vi "Random Color Generator.vi"(5 "Lightest Limit":u32(colorbox)=16448250, 7 "Darkest Limit":u32(colorbox), 11 "Color Exclude":u32[](array[colorbox])) -> (1 "Random Color":u32(colorbox), 3 "Color Exclude Out":u32[](array[numeric]))   [LabVIEW 2023]
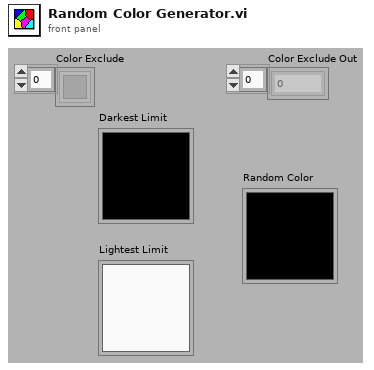
[diagram p1: front panel]
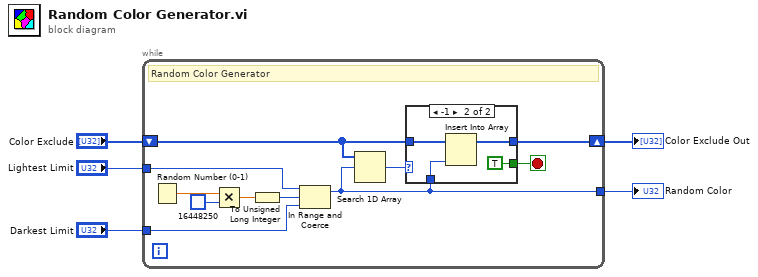
[diagram p0: block diagram]
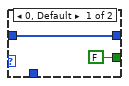
[diagram p2: hidden frame]
diagram:
  n1 = while {
    tunnel: "Darkest Limit" -> [w14]
    tunnel: "Lightest Limit" -> [w13]
    tunnel: [w8] -> w3
    shift-right: [w9] -> w1
    shift-left: "Color Exclude" -> [w10]
    stop <- w6 stop-if-true
    # "Random Color Generator"
    n2 = Random Number (0-1)() -> (number: 0 to 1=w16:dbl)
    n3 = Multiply(x=w16, y=u32 16448250 ("Lightest Limit 2")) -> (x*y=w12:dbl)
    n4 = To Unsigned Long Integer(number=w12) -> (unsigned 32bit integer=w11:u32)
    n5 = In Range and Coerce(upper limit=w13, x=w11, lower limit=w14) -> (coerced(x)=w8:u32)  [unwired: 1 out]
    n6 = Search 1D Array(1D array=w10, element=w8) -> (index of element=w7:i32)  [unwired: 1 in]
    n7 = case shown="-1" w7 {
      tunnel: w10 -> [w17 w22]
      tunnel: [w17 w21] -> w9
      tunnel: w8 -> [_ w20]
      tunnel: [FALSE TRUE] -> w6
      frame 0, Default {
      }
      frame -1 {
        n8 = Insert Into Array(array=w22, new element=w20) -> (w21:u32[])  [unwired: 1 in]
      }
    }
  }
  "Random Color" <- w3
  "Color Exclude Out" <- w1
